vi "4_2_MNIST_Inference(CPU)(RT).vi"() -> ()   [LabVIEW 2020]
doc: "This example demonstrates the usage of Deep Learning Toolkit for loading the model pretrained for handwritten digit recognition and running for inference on RT targets.\nRequirements: Deep Learning Toolkit for LabVIEW.\nMore Examples: https://github.com/ngenehub/deepltk_examples"
uses:
  <vilib>/Ngene/Deep Learning Toolkit/Toolkit/NN_Network/Controls/NN_Save_Before_Destroy_Options.ctl
  <vilib>/Ngene/Deep Learning Toolkit/Toolkit/NN_Network/API/NN_Set_Input/3D/NN_Set_Input(3D_SGL_idx).vi
  <vilib>/Ngene/Deep Learning Toolkit/Toolkit/Deep_Learning_Toolkit_by_Ngene.lvlib
  <vilib>/ptbypt/NI_PtbyPt.lvlib
panel:
  out "Labels":string[](array[string])=["0", "1", "2", "3", "4", "5", "6", "7", "8", "9"]
  in  "Stop":bool
  in  "Network Configuration File Path":path=path "D:/Ngene/GitHub/deepltk_fpga_examples/1_MNIST_Classification(PXI,sbRIO)/Models/0_Original/MNIST_CNN/MNIST_CNN_net_cfg_24_11_25__15_33_35.cfg"
  in  "Weight File Path":path=path "D:/Ngene/GitHub/deepltk_fpga_examples/1_MNIST_Classification(PXI,sbRIO)/Models/0_Original/MNIST_CNN/MNIST_CNN_weights_24_11_25__15_33_35.bin"
  out "Inference Speed (img/s)":dbl=42.94575461176154 format="%#_3p"
  out "Inference Time(s/img)":dbl=0.02328518870002881 format="%#_3p"
  out "Predictions":sgl[](array[slide])=[3.917579e-06, 8.7156375e-05, 1.1265606e-06, 1.5418425e-07, 0.9997638, 1.6421981e-06, 2.2499413e-05, 4.0262337e-05, 2.0309723e-09, 7.938153e-05] scale=0.0..1.0
  in  "Image (28x28px)":sgl[][](graph)=[[-1.0, -1.0, -1.0, -1.0, -1.0, -1.0, -1.0, -1.0, -1.0, -1.0, -1.0, -1.0, -1.0, -1.0, -1.0, -1.0, -1.0, -1.0, -1.0, -1.0, -1.0, -1.0, -1.0, -1.0, -1.0, -1.0, -1.0, -1.0], [-1.0, -1.0, -1.0, -1.0, -1.0, -1.0, -1.0, -1.0, -1.0, -1.0, -1.0, -1.0, -1.0, -1.0, -1.0, -1.0, -1.0, -1.0, -1.0, -1.0, -1.0, -1.0, -1.0, -1.0, -1.0, -1.0, -1.0, -1.0], [-1.0, -1.0, -1.0, -1.0, -1.0, -1.0, -1.0, -1.0, -1.0, -1.0, -1.0, -1.0, -1.0, -1.0, -1.0, -1.0, -1.0, -1.0, -1.0, -1.0, -1.0, -1.0, -1.0, -1.0, -1.0, -1.0, -1.0, -1.0], [-1.0, -1.0, -1.0, -1.0, -1.0, -1.0, -1.0, -1.0, -1.0, -1.0, -1.0, -1.0, -1.0, -1.0, -1.0, -1.0, -1.0, -1.0, -1.0, -1.0, -1.0, -1.0, -1.0, -1.0, -1.0, -1.0, -1.0, -1.0], [-1.0, -1.0, -1.0, -1.0, -1.0, -1.0, -1.0, -1.0, -0.7992126, 0.003937008, -0.6185039, -1.0, -1.0, -1.0, -1.0, -1.0, -1.0, -1.0, -1.0, -1.0, -1.0, -1.0, -1.0, -1.0, -1.0, -1.0, -1.0, -1.0], [-1.0, -1.0, -1.0, -1.0, -1.0, -1.0, -1.0, -1.0, 0.24488188, 1.007874, 0.5661417, -1.0, -1.0, -1.0, -1.0, -1.0, -1.0, -1.0, -1.0, -1.0, -1.0, -1.0, -1.0, -1.0, -1.0, -1.0, -1.0, -1.0], [-1.0, -1.0, -1.0, -1.0, -1.0, -1.0, -1.0, -1.0, 0.4055118, 1.007874, 0.42559054, -1.0, -1.0, -1.0, -1.0, -1.0, -1.0, -1.0, -1.0, -1.0, -1.0, -1.0, -1.0, -1.0, -1.0, -1.0, -1.0, -1.0], [-1.0, -1.0, -1.0, -1.0, -1.0, -1.0, -1.0, -1.0, 0.4055118, 1.007874, 0.4055118, -1.0, -1.0, -1.0, -1.0, -1.0, -1.0, -1.0, -1.0, -1.0, -1.0, -1.0, -1.0, -1.0, -1.0, -1.0, -1.0, -1.0], [-1.0, -1.0, -1.0, -1.0, -1.0, -1.0, -1.0, -1.0, 0.4055118, 1.007874, 0.4055118, -1.0, -1.0, -1.0, -1.0, -1.0, -1.0, -1.0, -1.0, -1.0, -1.0, -1.0, -1.0, -1.0, -1.0, -1.0, -1.0, -1.0], [-1.0, -1.0, -1.0, -1.0, -1.0, -1.0, -1.0, -1.0, 0.4055118, 1.007874, 0.4055118, -1.0, -1.0, -1.0, -1.0, -1.0, -1.0, -1.0, -1.0, -1.0, -1.0, -1.0, -1.0, -1.0, -1.0, -1.0, -1.0, -1.0], [-1.0, -1.0, -1.0, -1.0, -1.0, -1.0, -1.0, -1.0, 0.58622044, 1.007874, 0.32519686, -1.0, -1.0, -1.0, -1.0, -0.8393701, 0.78700787, 0.68661416, -0.91968507, -1.0, -1.0, -1.0, -1.0, -1.0, -1.0, -1.0, -1.0, -1.0], [-1.0, -1.0, -1.0, -1.0, -1.0, -1.0, -1.0, -1.0, 0.7468504, 1.007874, 0.16456693, -1.0, -1.0, -1.0, -1.0, -0.538189, 1.007874, 1.007874, -0.33740157, -1.0, -1.0, -1.0, -1.0, -1.0, -1.0, -1.0, -1.0, -1.0], [-1.0, -1.0, -1.0, -1.0, -1.0, -1.0, -1.0, -1.0, 0.9275591, 1.007874, -0.11653543, -1.0, -1.0, -1.0, -1.0, -0.9598425, 0.9275591, 1.007874, 0.28503937, -1.0, -1.0, -1.0, -1.0, -1.0, -1.0, -1.0, -1.0, -1.0], [-1.0, -1.0, -1.0, -1.0, -1.0, -1.0, -1.0, -0.87952757, 1.007874, 1.007874, -0.21692914, -1.0, -1.0, -1.0, -1.0, -1.0, 0.6062992, 1.007874, 0.82716537, -1.0, -1.0, -1.0, -1.0, -1.0, -1.0, -1.0, -1.0, -1.0], [-1.0, -1.0, -1.0, -1.0, -1.0, -1.0, -1.0, -0.7992126, 1.007874, 1.007874, -0.39763778, -1.0, -1.0, -1.0, -1.0, -1.0, 0.6062992, 1.007874, 1.007874, -0.91968507, -1.0, -1.0, -1.0, -1.0, -1.0, -1.0, -1.0, -1.0], [-1.0, -1.0, -1.0, -1.0, -1.0, -1.0, -1.0, -0.5984252, 1.007874, 1.007874, -0.4980315, -1.0, -1.0, -1.0, -1.0, -1.0, 0.70669293, 1.007874, 1.007874, -0.5582677, -1.0, -1.0, -1.0, -1.0, -1.0, -1.0, -1.0, -1.0], [-1.0, -1.0, -1.0, -1.0, -1.0, -1.0, -1.0, -0.5984252, 1.007874, 1.007874, 0.5259842, 0.4055118, 0.4055118, 0.4055118, 0.4055118, 0.48582676, 1.007874, 1.007874, 1.007874, -0.13661417, -1.0, -1.0, -1.0, -1.0, -1.0, -1.0, -1.0, -1.0], [-1.0, -1.0, -1.0, -1.0, -1.0, -1.0, -1.0, -0.8393701, 0.9476378, 1.007874, 1.007874, 1.007874, 1.007874, 1.007874, 1.007874, 1.007874, 1.007874, 1.007874, 1.007874, -0.07637795, -1.0, -1.0, -1.0, -1.0, -1.0, -1.0, -1.0, -1.0], [-1.0, -1.0, -1.0, -1.0, -1.0, -1.0, -1.0, -1.0, -0.2972441, 0.4055118, 0.4055118, 0.4055118, 0.4055118, 0.4055118, 0.4055118, 0.34527558, -0.036220472, 1.007874, 1.007874, -0.17677166, -1.0, -1.0, -1.0, -1.0, -1.0, -1.0, -1.0, -1.0], [-1.0, -1.0, -1.0, -1.0, -1.0, -1.0, -1.0, -1.0, -1.0, -1.0, -1.0, -1.0, -1.0, -1.0, -1.0, -1.0, -1.0, 0.8070866, 1.007874, 0.003937008, -1.0, -1.0, -1.0, -1.0, -1.0, -1.0, -1.0, -1.0], [-1.0, -1.0, -1.0, -1.0, -1.0, -1.0, -1.0, -1.0, -1.0, -1.0, -1.0, -1.0, -1.0, -1.0, -1.0, -1.0, -1.0, 0.8070866, 1.007874, 0.14448819, -1.0, -1.0, -1.0, -1.0, -1.0, -1.0, -1.0, -1.0], [-1.0, -1.0, -1.0, -1.0, -1.0, -1.0, -1.0, -1.0, -1.0, -1.0, -1.0, -1.0, -1.0, -1.0, -1.0, -1.0, -1.0, 0.72677165, 1.007874, 0.14448819, -1.0, -1.0, -1.0, -1.0, -1.0, -1.0, -1.0, -1.0], [-1.0, -1.0, -1.0, -1.0, -1.0, -1.0, -1.0, -1.0, -1.0, -1.0, -1.0, -1.0, -1.0, -1.0, -1.0, -1.0, -1.0, 0.6062992, 1.007874, 0.26496062, -1.0, -1.0, -1.0, -1.0, -1.0, -1.0, -1.0, -1.0], [-1.0, -1.0, -1.0, -1.0, -1.0, -1.0, -1.0, -1.0, -1.0, -1.0, -1.0, -1.0, -1.0, -1.0, -1.0, -1.0, -1.0, 0.6062992, 1.007874, 0.32519686, -1.0, -1.0, -1.0, -1.0, -1.0, -1.0, -1.0, -1.0], [-1.0, -1.0, -1.0, -1.0, -1.0, -1.0, -1.0, -1.0, -1.0, -1.0, -1.0, -1.0, -1.0, -1.0, -1.0, -1.0, -1.0, 0.6062992, 1.007874, 0.20472442, -1.0, -1.0, -1.0, -1.0, -1.0, -1.0, -1.0, -1.0], [-1.0, -1.0, -1.0, -1.0, -1.0, -1.0, -1.0, -1.0, -1.0, -1.0, -1.0, -1.0, -1.0, -1.0, -1.0, -1.0, -1.0, 0.6062992, 1.007874, 0.20472442, -1.0, -1.0, -1.0, -1.0, -1.0, -1.0, -1.0, -1.0], [-1.0, -1.0, -1.0, -1.0, -1.0, -1.0, -1.0, -1.0, -1.0, -1.0, -1.0, -1.0, -1.0, -1.0, -1.0, -1.0, -1.0, 0.08425197, 1.007874, -0.11653543, -1.0, -1.0, -1.0, -1.0, -1.0, -1.0, -1.0, -1.0], [-1.0, -1.0, -1.0, -1.0, -1.0, -1.0, -1.0, -1.0, -1.0, -1.0, -1.0, -1.0, -1.0, -1.0, -1.0, -1.0, -1.0, -1.0, -0.81929135, -1.0, -1.0, -1.0, -1.0, -1.0, -1.0, -1.0, -1.0, -1.0]]
  # "Overview: This example demonstrates the usage of Deep Learning Toolkit for loading the model pretrained for handwritten digit recognition and running for inference on RT targets.\nRequirements: \nDeepLTK - Deep Learning Toolkit for LabVIEW (https://www.ngene.co/deep-learning-toolkit-for-labview)\nInstructions:\nThis example runs in parallel with \"4_1_MNIST_Drawing_Interface(CPU).vi\", which is required to generate test samples.\n1.\tCopy the pretrained model generated by \"0_MNIST(Train).vi\" to the RT target.\n2.\tProvide paths to .cfg and .bin files located on the RT target at \"Network Configuration File Path\" and \"Weight File Path\" controls.\n3.\tRun the VI.\n4.\tDraw a digit in \"Drawing_Interface(Host).vi\" and copy data from \"Image (28x28px)\".\n5.\tRight click on \"Image (28x28px)\" on this VI and select \"Paste Data\".\n6.\tObserve \"Predictions\" results and inference speed/time.\nMore Examples:  https://github.com/ngenehub/deepltk_examples"
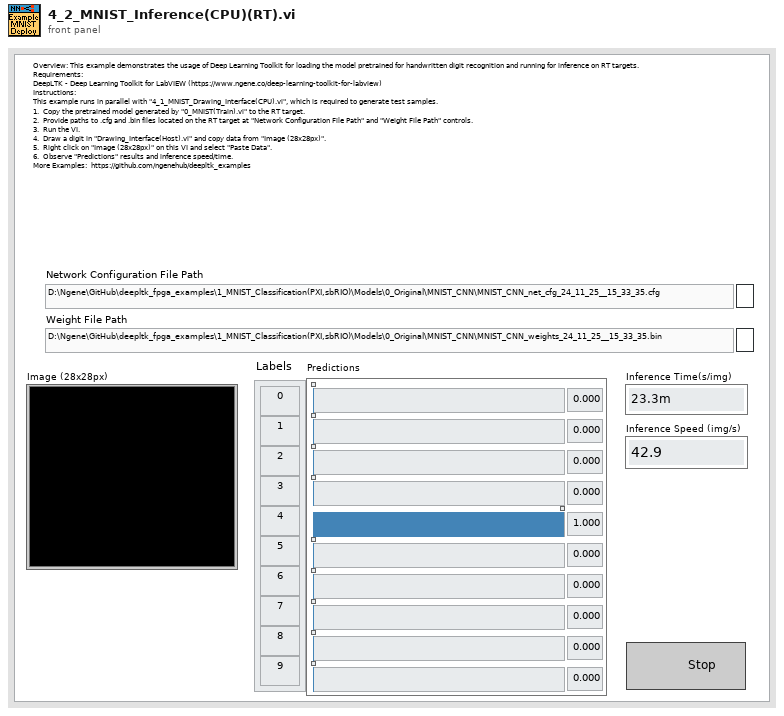
[diagram p1: front panel]
types:
  T1 = typedef "Deep_Learning_Toolkit_by_Ngene.lvlib/NN_Save_Before_Destroy_Options.ctl" = cluster{"CFG?":bool, "Weights?":bool, "Render?":bool}
  T2 = typedef "Deep_Learning_Toolkit_by_Ngene.lvlib/NN_Config_Params.ctl" = cluster{"Name":string, "mBatch":i32, "NN_Train_Params":T3, "LR_Decay_Policy":T6, "Labels":string[], "Loss":T8}
  T3 = typedef "Deep_Learning_Toolkit_by_Ngene.lvlib/NN_Train_Params.ctl" = cluster{"Optimizer":T4, "Beta_1":sgl, "Beta_2":sgl, "Weight Decay(L1)":sgl, "Weight Decay(L2)":sgl, "Data_Sampling":T5}
  T4 = typedef "Deep_Learning_Toolkit_by_Ngene.lvlib/NN_Train_Optimizer.ctl" = enum16{"SGD", "Adam", "Adagrad", "Adadelta", "RMSProp", "Nesterov"}
  T5 = typedef "Deep_Learning_Toolkit_by_Ngene.lvlib/NN_Train_Data_Sampling.ctl" = enum16{"Random", "Sequential"}
  T6 = typedef "Deep_Learning_Toolkit_by_Ngene.lvlib/NN_LR_Policy_Cfg.ctl" = cluster{"Policy_Type":T7, "LR0":dbl, "k":sgl, "WarmUp_Policy":enum16{"Step", "Ramp"}, "WarmUp_Iter":i32, "WarmUp_Ratio":sgl}
  T7 = typedef "Deep_Learning_Toolkit_by_Ngene.lvlib/NN_LR_Policy_Type.ctl" = enum16{"Manual", "Step", "Exp", "1/t"}
  T8 = typedef "Deep_Learning_Toolkit_by_Ngene.lvlib/NN_Loss_Config_Params.ctl" = cluster{"Loss_Type":T9, "Loss_Conf_Params":variant}
  T9 = typedef "Deep_Learning_Toolkit_by_Ngene.lvlib/NN_Loss_Type.ctl" = enum16{"None", "MSE", "CrossEntropy", "YOLO_v2", "YOLO_v4"}
  T10 = typedef "Deep_Learning_Toolkit_by_Ngene.lvlib/NN_Layer_Config_Params.ctl" = cluster{"Layer_Type":T11, "Layer_Conf_Params":variant, "Input Layers":string[]}
  T11 = typedef "Deep_Learning_Toolkit_by_Ngene.lvlib/NN_Layer_Type.ctl" = enum16{"Input1D", "Input3D", "Conv1D", "Conv2D", "Conv2D_Adv", "MaxPool", "AvgPool", "UpSample", "DropOut3D", "ShortCut", "Concat", "SoftMax3D", "FC", "DropOut", "Softmax", "Flatten", "YOLO_v2", "YOLO_v4", "Activation", "BatchNormalization", "Unsupported"}
  T12 = typedef "Deep_Learning_Toolkit_by_Ngene.lvlib/NN.ctl" = cluster{"Name":string, "No of Layers":i32, "mBatch":i32, "Layers":T13[], "Dimty":T14, "Dims_In":T15, "Dims_Out":T15, "Working_Dir":path, "Train?":bool, "Train_Params":T3, "LR_Update_Policy":T6, "Session Data":T16, "Ground_truth":T17, "NNg_hdls":T18, "NN_Device":T19, "GPU Id":i32, "Labels":string[], "Receptive Field":T20[], "Loss_Type":T9, "Loss_Cfg_Prms":variant, "NNG_WS":T21}
  T13 = typedef "Deep_Learning_Toolkit_by_Ngene.lvlib/NN_Layer_ref.ctl" = refnum<data-value>
  T14 = typedef "Deep_Learning_Toolkit_by_Ngene.lvlib/NN_In_Out_Dim-ty.ctl" = enum8{"In1D_Out1D", "In3D_Out1D", "In3D_Out3D", "In3D_OutBBox"}
  T15 = typedef "Deep_Learning_Toolkit_by_Ngene.lvlib/NN_Dims(C,H,W).ctl" = cluster{"C":i32, "H":i32, "W":i32}
  T16 = typedef "Deep_Learning_Toolkit_by_Ngene.lvlib/NN_Train_Session_Data.ctl" = cluster{"Epochs":sgl, "Tot_Iter":i32, "LR":sgl, "LR_iter":i32}
  T17 = typedef "Deep_Learning_Toolkit_by_Ngene.lvlib/NN_Ground_truth.ctl" = cluster{"Y":variant}
  T18 = typedef "Deep_Learning_Toolkit_by_Ngene.lvlib/nng_cuda_handles.ctl" = cluster{"cudnn":u64, "cublas":u64, "stream":u64, "curand":u64}
  T19 = typedef "Deep_Learning_Toolkit_by_Ngene.lvlib/NN_Device.ctl" = enum16{"CPU", "GPU"}
  T20 = typedef "Deep_Learning_Toolkit_by_Ngene.lvlib/NN_Dims(V,H).ctl" = cluster{"V":i32, "H":i32}
  T21 = typedef "Deep_Learning_Toolkit_by_Ngene.lvlib/NNG_WS.ctl" = cluster{"NNG_WS_Mem":T22, "Max_WS_Size":i64}
  T22 = typedef "Deep_Learning_Toolkit_by_Ngene.lvlib/NNg_WS_Mem_DVR.ctl" = refnum<data-value>
  T23 = typedef "Deep_Learning_Toolkit_by_Ngene.lvlib/NN_Layer.ctl" = cluster{"Name":string, "Layer_Data":variant, "Layer_Type":T11, "Dims_In":T15, "Layers_In":variant, "Dims_Out":T15, "Layers_Out":variant, "Metrics":T24, "GPU_Data":variant, "mBatch":i32, "NN_Device":T19, "NNg_hdls":T18, "Train?":bool, "Dimty":T25, "RecptField":T26}
  T24 = typedef "Deep_Learning_Toolkit_by_Ngene.lvlib/NN_Layer_Metrics.ctl" = cluster{"Data":dbl, "Params":dbl, "Ops":dbl}
  T25 = typedef "Deep_Learning_Toolkit_by_Ngene.lvlib/NN_Layer_Dimty.ctl" = enum16{"1D", "3D"}
  T26 = typedef "Deep_Learning_Toolkit_by_Ngene.lvlib/NN_Layer_RF_State.ctl" = cluster{"Dims":T20, "J":T20}
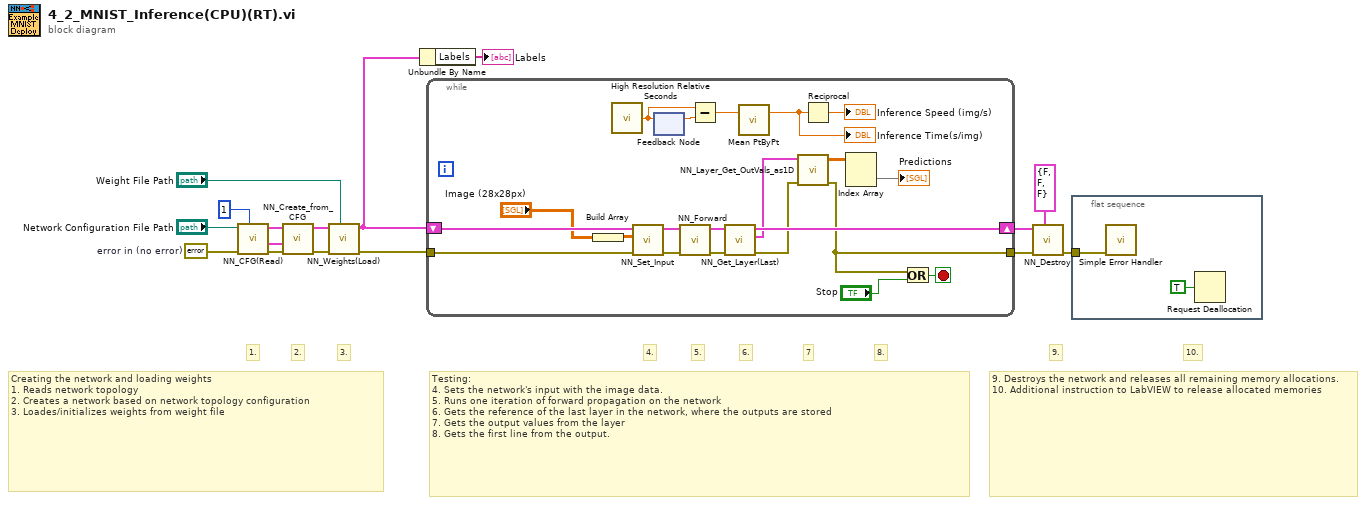
[diagram p0: block diagram]
diagram:
  w9 = errorcluster {"status"=FALSE, "code"=0, "source"=""}  # error in (no error)
  # "9.\tDestroys the network and releases all remaining memory allocations.\n10.\tAdditional instruction to LabVIEW to release allocated memories"
  # "Creating the network and loading weights\n1.\tReads network topology\n2.\tCreates a network based on network topology configuration\n3.\tLoades/initializes weights from weight file"
  # "3."
  # "2."
  # "1."
  # "10."
  # "9."
  # "Testing: \n4.\tSets the network's input with the image data.\n5.\tRuns one iteration of forward propagation on the network\n6.\tGets the reference of the last layer in the network, where the outputs are stored\n7.\tGets the output values from the layer\n8.\tGets the first line from the output."
  # "8."
  # "7"
  # "6."
  # "5."
  # "4."
  n1 = call <vilib>:"NN_CFG(Read).vi"("mBatch"=1, "error in (no error)"=w9, "CFG file path"="Network Configuration File Path") -> ("error out"=w7:errorcluster, "Net_Cfg"=w8:T2, "Layer_Cfg"=w6:T10[])  [unwired: 6 in]
  n2 = call <vilib>:"NN_Create_from_CFG.vi"("error in (no error)"=w7, "Net_Cfg"=w8, "Layer_Cfg"=w6) -> ("error out"=w11:errorcluster, "NN out"=w5:T12)  [unwired: 7 in]
  n3 = call <vilib>:"NN_Weights(Load).vi"("Weight File Path"="Weight File Path", "error in (no error)"=w11, "NN in"=w5) -> ("error out"=w4:errorcluster, "NN out"=w2:T12)  [unwired: 7 in]
  n4 = Unbundle By Name(w2) -> ("Labels"=→"Labels":string[])
  n5 = while {
    shift-right: [w36] -> w15
    shift-left: w2 -> [w29]
    tunnel: w4 -> [w27]
    tunnel: [w21] -> w14
    stop <- w34 stop-if-true
    n6 = Build Array("Image (28x28px)") -> (w20:sgl[][][])
    n7 = call <vilib>:"High Resolution Relative Seconds.vi"() -> ("relative seconds"=w32:dbl)
    n8 = call-poly <vilib>:"NN_Set_Input.vi"("error in (no error)"=w27, "Data_In(3D_SGL)"=w20, "NN in"=w29) -> ("error out"=w26:errorcluster, "NN out"=w28:T12)  [unwired: 7 in]
    n9 = feedback #1() -> (w33:dbl)  [unwired: 1 in]
    n10 = feedback-in #1(w32) -> ()
    n11 = call <vilib>:"NN_Forward.vi"("error in (no error)"=w26, "NN in"=w28) -> ("error out"=w35:errorcluster, "NN out"=w37:T12)  [unwired: 6 in, 2 out]
    n12 = Subtract(x=w32, y=w33) -> (x-y=w31:dbl)
    n13 = call <vilib>:"NN_Get_Layer(Last).vi"("error in (no error)"=w35, "NN in"=w37) -> ("error out"=w22:errorcluster, "Last_Layer"=w25:T23, "NN out"=w36:T12)  [unwired: 6 in, 1 out]
    n14 = call <vilib>:"Mean PtByPt.vi"("x"=w31) -> ("mean"=w17:dbl)  [unwired: 3 in, 1 out]
    "Inference Time(s/img)" <- w17
    n15 = call <vilib>:"NN_Layer_Get_OutVals_as1D.vi"("error in (no error)"=w22, "Layer"=w25) -> ("error out"=w21:errorcluster, "Out(as1D)"=w24:sgl[][])  [unwired: 8 in]
    n16 = Reciprocal(x=w17) -> (1/x=→"Inference Speed (img/s)":dbl)
    n17 = Index Array(array=w24) -> (element=→"Predictions":sgl[])  [unwired: 2 in]
    n18 = Or(x=w21, y="Stop") -> (x .or. y?=w34:bool)
  }
  n19 = call <vilib>:"NN_Destroy.vi"("Save (T, T, T)"=T1 {"CFG?"=FALSE, "Weights?"=FALSE, "Render?"=FALSE} ("Save_Config"), "error in (no error)"=w14, "NN in"=w15) -> ("error out"=w16:errorcluster)  [unwired: 7 in, 1 out]
  n20 = flat-sequence {
    tunnel: w16 -> [w39]
    frame #0 {
      n21 = call <vilib>:"Simple Error Handler.vi"("error in (no error)"=w39) -> ()  [unwired: 4 in, 5 out]
      n22 = Request Deallocation(TRUE ("flag")) -> ()
    }
  }
